vi "SVPO RMS Level (N Ch DBL WDT).vi"(6 "restart averaging? (F)":bool, 11 "scaled signals [EU]":waveform(dbl)[](array[waveform])) -> (3 "RMS levels":dbl[](array[numeric]), 4 "durations [s]":dbl[](array[numeric]), 5 "timestamps":timestamp[](array[timestamp]))   [LabVIEW 2017, in "SoundVib_VibrationLevel.lvlib"]
doc: "Computes the root-mean-square (RMS) level of scaled time waveform signals and scaled array signals. <B>scaled signal [EU]</B> should have a zero DC component. You can attenuate the DC component with hardware AC-coupling filters and with software high-pass filters. Use this VI on embedded targets that have limited computational resources. Wire data to the <B>scaled signal [EU]</B> input to determine the polymorphic instance to use or manually select the instance."
uses:
  <vilib>/addons/Sound and Vibration/svt_Level/SoundVib_VibrationLevel.lvlib
  <vilib>/addons/_NISVFA/_Shared subVIs/Controls/svc_RMS Level State.ctl
  <vilib>/addons/Sound and Vibration/svt_Level/SVPO RMS Level (1 Ch DBL Array) with IC.vi
  <vilib>/Analysis/baseanly.llb/Dot Product.vi
  <vilib>/Analysis/baseanly.llb/Real Dot Product.vi
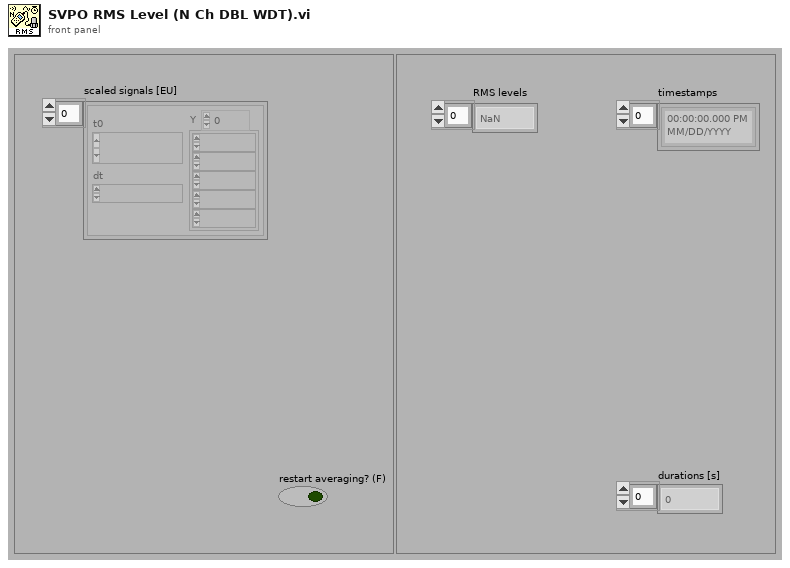
[diagram p1: front panel]
types:
  T1 = typedef "svc_RMS Level State.ctl" = cluster{"Squared Sum":dbl, "Size":u64, "timestamp":timestamp}
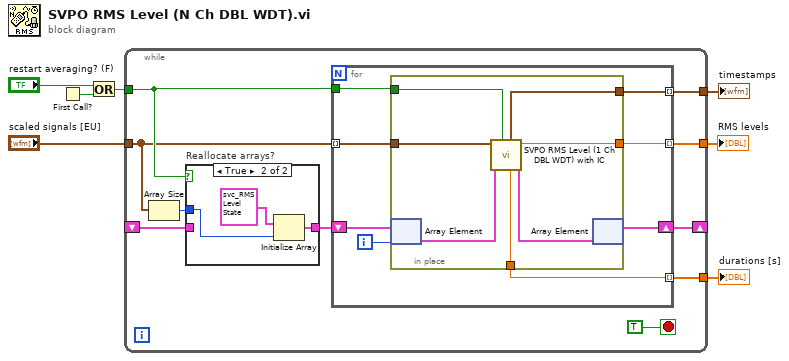
[diagram p0: block diagram]
diagram:
  n1 = First Call?() -> (First Call?: T/F=w7:bool)
  n2 = Or(x="restart averaging? (F)", y=w7) -> (x .or. y?=w5:bool)
  n3 = while {
    tunnel: w5 -> [w12]
    tunnel: "scaled signals [EU]" -> [w9]
    tunnel: [w16] -> w3
    shift-right: [w14] -> _
    shift-left: _ -> [w13]
    tunnel: [w11] -> w2
    tunnel: [w10] -> w1
    stop <- TRUE stop-if-true
    n4 = Array Size(array=w9) -> (size(s)=w8:i32)
    n5 = case "Reallocate arrays?" shown="True" w12 {
      tunnel: [w18 w21] -> w15
      tunnel: w13 -> [w18 _]
      tunnel: w8 -> [_ w19]
      frame False {
      }
      frame True {
        n6 = Initialize Array(T1 {"Squared Sum"=0.0, "Size"=0, "timestamp"=timestamp(0 s since 1904-01-01)} ("Initial Conditions"), w19) -> (w21:T1[])
      }
    }
    n7 = for {
      tunnel: w9 -> [w29] mode=indexing
      tunnel: w12 -> [w23]
      tunnel: [w25] -> w16 mode=indexing
      shift-right: [w22] -> w14
      shift-left: w15 -> [w28]
      tunnel: [w26] -> w11 mode=indexing
      tunnel: [w24] -> w10 mode=indexing
      i -> [w27]
      n8 = in-place {
        in-place-border: w29 -> [w36]
        in-place-border: [w35] -> w26
        in-place-border: [w32] -> w25
        in-place-border: [w31] -> w24
        in-place-border: w23 -> [w30]
        n9 = in-place-array #1(w28, w27) -> (w34:T1)
        n10 = call <vilib>:"SVPO RMS Level (1 Ch DBL WDT) with IC.vi"("restart averaging? (F)"=w30, "initial conditions"=w34, "scaled signal [EU]"=w36) -> ("final conditions"=w33:T1, "RMS level"=w31:dbl, "duration [s]"=w32:dbl, "timestamp"=w35:timestamp)  [unwired: 5 in]
        n11 = in-place-array #1(w33) -> (w22:T1[])  [unwired: 1 out]
      }
    }
  }
  "RMS levels" <- w1
  "timestamps" <- w2
  "durations [s]" <- w3
